vi "Define DataTable Columns.vi"(8 "error in (no error)":errorcluster, 10 "ColumnSetup":T1[](array[typedef]) {"MinWidth" min=2 step=1; "AutoSizeMode" items=["None"=1, "ColumnHeader"=2, "AllCellsExceptHeader"=4, "AllCells"=6, "DisplayedCellsExceptHeader"=8, "DisplayedCells"=10, "Fill"=16]; "FillWeight" min=1 max=100}, 11 "DataTable In":refnum<class "DataTable.lvclass">) -> (0 "error out":errorcluster, 3 "DataTable Out":refnum<class "DataTable.lvclass">)   [LabVIEW 2013, in "DataGrid.lvlib" / "DataTable.lvclass"]
doc: "Defines the columns of the dataTable that is used to store all display data. If called more than once, it will add columns to the existing dataTable, so resulting in more (possibly duplicate) columns."
uses:
  DataTable/DataTable.lvclass
  GridColumn/ColumnDefinition.ctl
  GridColumn/ColumnType.ctl
  DataTable/DataTable.lvclass/DataTable.ctl
  System.Data
  DataTable/Read DataTable.vi
  GridColumn/GridColumn.lvclass
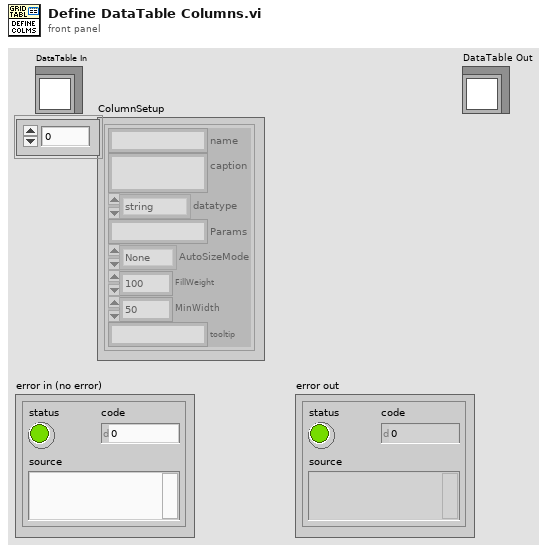
[diagram p1: front panel]
types:
  T1 = typedef "DataGrid.lvlib/GridColumn.lvclass/ColumnDefinition.ctl" = cluster{"name":string, "caption":string, "datatype":T2, "Params":string, "AutoSizeMode":i32, "FillWeight":sgl, "MinWidth":u32, "tooltip":string}
  T2 = typedef "DataGrid.lvlib/GridColumn.lvclass/ColumnType.ctl" = enum16{"string", "image", "check", "numeric", "timestamp", "button", "combo", "link"}
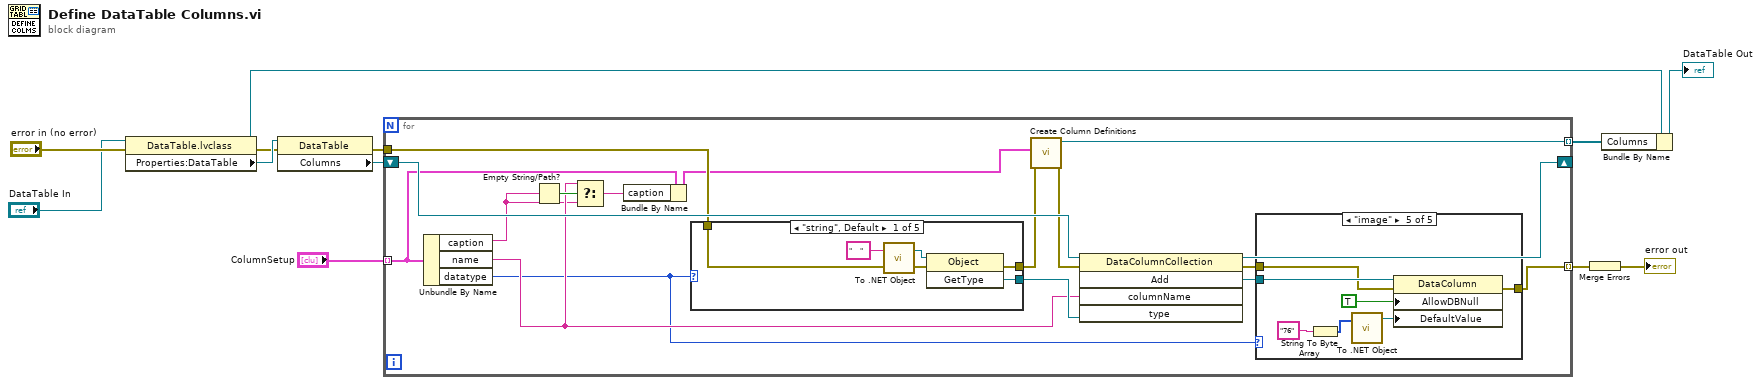
[diagram p0: block diagram]
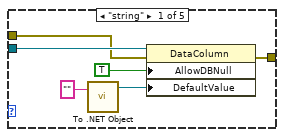
[diagram p2: hidden frame]
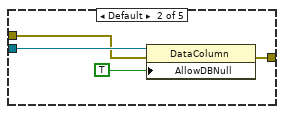
[diagram p3: hidden frame]
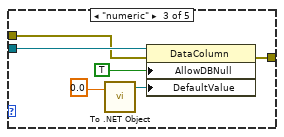
[diagram p4: hidden frame]
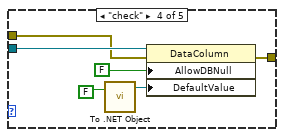
[diagram p5: hidden frame]
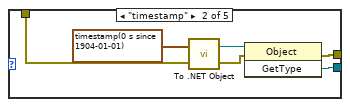
[diagram p6: hidden frame]
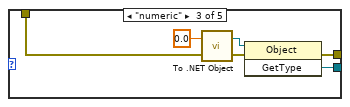
[diagram p7: hidden frame]
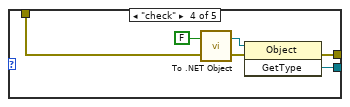
[diagram p8: hidden frame]
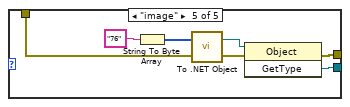
[diagram p9: hidden frame]
diagram:
  n1 = property class="DataTable.lvclass"(reference="DataTable In", error in="error in (no error)") -> (reference out=w3:refnum<class "DataTable.lvclass">, error out=w6:errorcluster, "Properties:DataTable"=w8:refnum<k24>)
  n2 = property class="DataTable"(reference=w8, error in=w6) -> (error out=w5:errorcluster, "Columns"=w7:refnum<k24>)  [unwired: 1 out]
  n3 = for {
    tunnel: "ColumnSetup" -> [w20] mode=indexing
    tunnel: [w14] -> w10 mode=indexing
    shift-right: [w17] -> _
    shift-left: w7 -> [w29]
    tunnel: [w27] -> w1 mode=indexing
    tunnel: w5 -> [w26]
    n4 = Unbundle By Name(w20) -> ("caption"=w18:string, "name"=w22:string, "datatype"=w13:T2)
    n5 = Empty String/Path?(string/path=w18) -> (empty?=w23:bool)
    n6 = Select(t=w22, s=w23, f=w18) -> (s? t:f=w21:string)
    n7 = Bundle By Name(cluster=w20, "caption"=w21) -> (w19:T1)
    n8 = case shown="\"string\", Default" w13 {
      tunnel: [w62 w68 w72 w80 w86] -> w28
      tunnel: [w61 w66 w73 w79 w84] -> w25
      tunnel: w26 -> [w59 w65 w71 w77 w83]
      frame "string", Default {
        n9 = call <vilib>:"To .NET Object.vi"("error in (no error)"=w59, "anything"="    " ("name")) -> ("error out"=w60:errorcluster, ".NET object"=w63:refnum<k24>)
        n10 = invoke class="Object" method="GetType"(reference=w63, error in=w60) -> (error out=w61:errorcluster, "GetType"=w62:refnum<k24>)  [unwired: 1 in, 1 out]
      }
      frame "timestamp" {
        n11 = call <vilib>:"To .NET Object.vi"("error in (no error)"=w65, "anything"=timestamp(0 s since 1904-01-01) ("name")) -> ("error out"=w67:errorcluster, ".NET object"=w69:refnum<k24>)
        n12 = invoke class="Object" method="GetType"(reference=w69, error in=w67) -> (error out=w66:errorcluster, "GetType"=w68:refnum<k24>)  [unwired: 1 in, 1 out]
      }
      frame "numeric" {
        n13 = call <vilib>:"To .NET Object.vi"("error in (no error)"=w71, "anything"=0.0 ("name")) -> ("error out"=w74:errorcluster, ".NET object"=w75:refnum<k24>)
        n14 = invoke class="Object" method="GetType"(reference=w75, error in=w74) -> (error out=w73:errorcluster, "GetType"=w72:refnum<k24>)  [unwired: 1 in, 1 out]
      }
      frame "check" {
        n15 = call <vilib>:"To .NET Object.vi"("error in (no error)"=w77, "anything"=FALSE) -> ("error out"=w78:errorcluster, ".NET object"=w82:refnum<k24>)
        n16 = invoke class="Object" method="GetType"(reference=w82, error in=w78) -> (error out=w79:errorcluster, "GetType"=w80:refnum<k24>)  [unwired: 1 in, 1 out]
      }
      frame "image" {
        n17 = String To Byte Array(string="76") -> (unsigned byte array=w88:u8[])
        n18 = call <vilib>:"To .NET Object.vi"("error in (no error)"=w83, "anything"=w88) -> ("error out"=w85:errorcluster, ".NET object"=w89:refnum<k24>)
        n19 = invoke class="Object" method="GetType"(reference=w89, error in=w85) -> (error out=w84:errorcluster, "GetType"=w86:refnum<k24>)  [unwired: 1 in, 1 out]
      }
    }
    n20 = call "Create Column Definitions.vi"("error in (no error)"=w25, "Column"=w19) -> ("error out"=w24:errorcluster, "GridColumn out"=w27:refnum<class "GridColumn.lvclass">)  [unwired: 8 in]
    n21 = invoke class="DataColumnCollection" method="Add"(reference=w29, error in=w24, "columnName"=w22, "type"=w28) -> (reference out=w17:refnum<k24>, error out=w15:errorcluster, "Add"=w16:refnum<k24>)  [unwired: 1 in, 2 out]
    n22 = case shown="\"image\"" w13 {
      tunnel: w16 -> [w35 w39 w45 w51 w58]
      tunnel: w15 -> [w34 w38 w44 w50 w57]
      tunnel: [w33 w37 w43 w49 w56] -> w14
      frame "string" {
        n23 = call <vilib>:"To .NET Object.vi"("anything"="" ("name")) -> (".NET object"=w30:refnum<k24>)  [unwired: 1 in, 1 out]
        n24 = property class="DataColumn"(reference=w35, error in=w34, "AllowDBNull"=TRUE, "DefaultValue"=w30) -> (error out=w33:errorcluster)  [unwired: 1 out]
      }
      frame Default {
        n25 = property class="DataColumn"(reference=w39, error in=w38, "AllowDBNull"=TRUE) -> (error out=w37:errorcluster)  [unwired: 1 out]
      }
      frame "numeric" {
        n26 = call <vilib>:"To .NET Object.vi"("anything"=0.0) -> (".NET object"=w41:refnum<k24>)  [unwired: 1 in, 1 out]
        n27 = property class="DataColumn"(reference=w45, error in=w44, "AllowDBNull"=TRUE, "DefaultValue"=w41) -> (error out=w43:errorcluster)  [unwired: 1 out]
      }
      frame "check" {
        n28 = call <vilib>:"To .NET Object.vi"("anything"=FALSE ("AllowDBNull")) -> (".NET object"=w47:refnum<k24>)  [unwired: 1 in, 1 out]
        n29 = property class="DataColumn"(reference=w51, error in=w50, "AllowDBNull"=FALSE, "DefaultValue"=w47) -> (error out=w49:errorcluster)  [unwired: 1 out]
      }
      frame "image" {
        n30 = String To Byte Array(string="76") -> (unsigned byte array=w52:u8[])
        n31 = call <vilib>:"To .NET Object.vi"("anything"=w52) -> (".NET object"=w54:refnum<k24>)  [unwired: 1 in, 1 out]
        n32 = property class="DataColumn"(reference=w58, error in=w57, "AllowDBNull"=TRUE, "DefaultValue"=w54) -> (error out=w56:errorcluster)  [unwired: 1 out]
      }
    }
  }
  n33 = Merge Errors(w10) -> (→"error out":errorcluster)
  n34 = Bundle By Name(cluster=w3, "Columns"=w1) -> (→"DataTable Out":refnum<class "DataTable.lvclass">)
